vi "status code of previous command.vi"() -> ()   [LabVIEW 2009]
panel:
  out "Display (F:Off)":bool
  out "dup VISA session":refnum<visa-resource-name>
  in  "VISA session":refnum<visa-resource-name>
  out "error out":errorcluster
  in  "error in (no error)":errorcluster
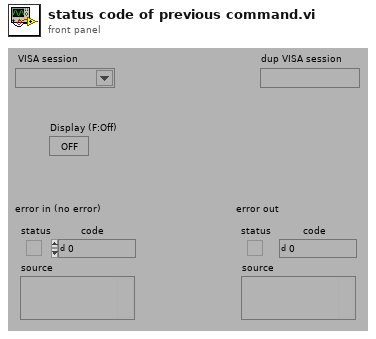
[diagram p1: front panel]
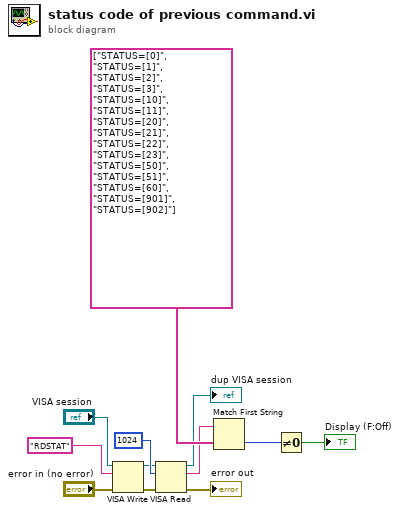
[diagram p0: block diagram]
diagram:
  n1 = VISA Write(VISA resource name="VISA session", write buffer="RDSTAT", error in (no error)="error in (no error)") -> (VISA resource name out=w5:refnum<visa-resource-name>, error out=w6:errorcluster)  [unwired: 1 out]
  n2 = VISA Read(VISA resource name=w5, byte count=u32 1024 ("byte count (0)"), error in (no error)=w6) -> (VISA resource name out=→"dup VISA session":refnum<visa-resource-name>, read buffer=w8:string, error out=→"error out":errorcluster)  [unwired: 1 out]
  n3 = Match First String(2:string[] ["STATUS=[0]", "STATUS=[1]", "STATUS=[2]", "STATUS=[3]", "STATUS=[10]", "STATUS=[11]", "STATUS=[20]", "STATUS=[21]", "STATUS=[22]", "STATUS=[23]", "STATUS=[50]", "STATUS=[51]", "STATUS=[60]", "STATUS=[901]", "STATUS=[902]"] ("string array"), 3:w8) -> (0:w7:i32)  [unwired: 1 out]
  n4 = Not Equal To 0?(x=w7) -> (x != 0?=→"Display (F:Off)":bool)
